vi "FGV_SerialControl.vi"(0 "Action":T1=enum."Close Serial Port", 1 "VISA Refnum in":refnum<visa-resource-name>="COM6", 2 "Channel":u8=255 step=1, 3 "Voltage":dbl min=0.0 max=4095.0 step=1.0, 4 "Wait Time (ms)":u32=4) -> (7 "VISA Refnum out":refnum<visa-resource-name>, 8 "Channels":u8[](array[numeric]), 9 "Voltages":u16[](array[numeric]), 10 "error out":errorcluster={"status"=FALSE, "code"=1073676294, "source"="VISA Read in SVI_ReadFromArduino.vi->FGV_SerialControl.vi->DemoForLoopWriteRead.vi"})   [LabVIEW 2020]
uses:
  Typedef_SerialFGVActions.ctl
  <vilib>/Instr/_visa.llb/VISA Configure Serial Port (Instr).vi
panel:
  out "Connection time (ms)":u32=1460
  out "read buffer":string="Connected\r\n"
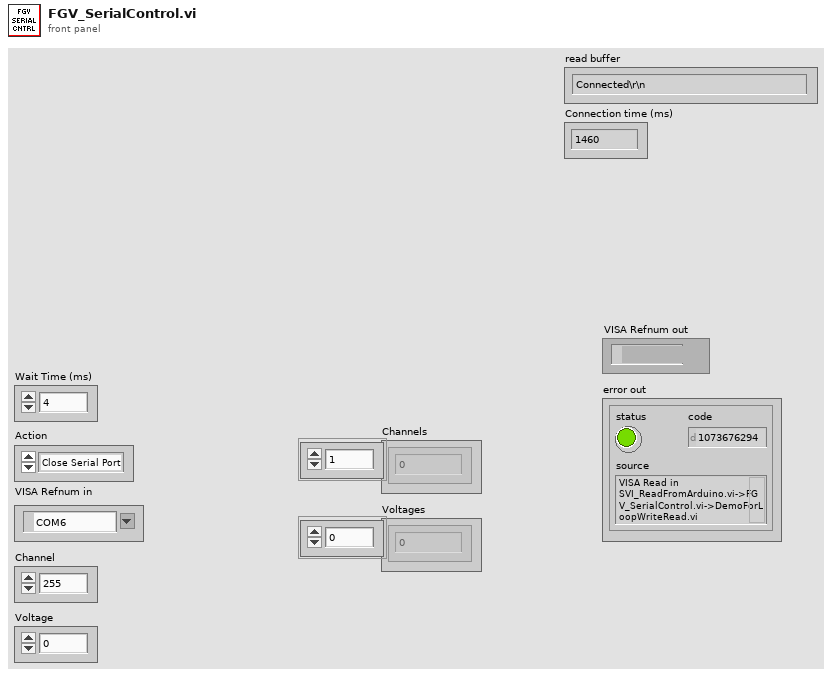
[diagram p1: front panel]
types:
  T1 = typedef "Typedef_SerialFGVActions.ctl" = enum16{"Open Serial Port", "Close Serial Port", "Update DAC", "Read ADC", "Read All ADCs"}
  T2 = cluster{"baud rate":u32, "data bits":u16, "parity":enum16{"None", "Odd", "Even", "Mark", "Space"}, "stop bits":u16, "flow control":u16}
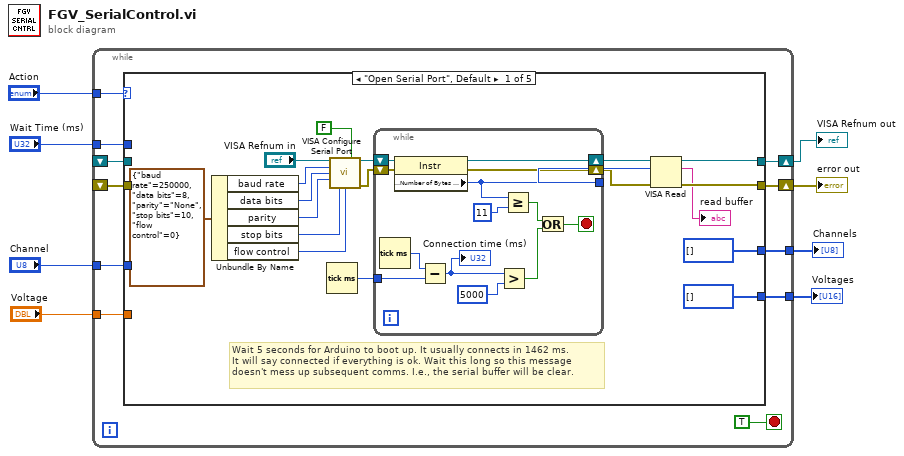
[diagram p0: block diagram]
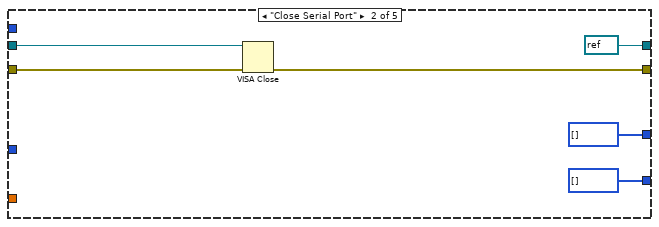
[diagram p2: hidden frame]
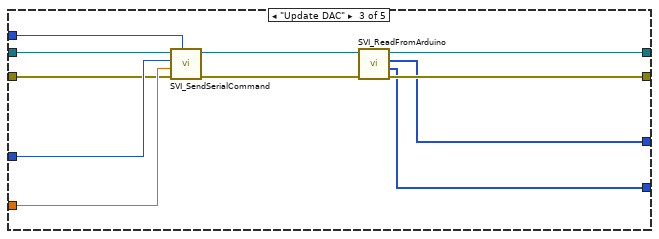
[diagram p3: hidden frame]
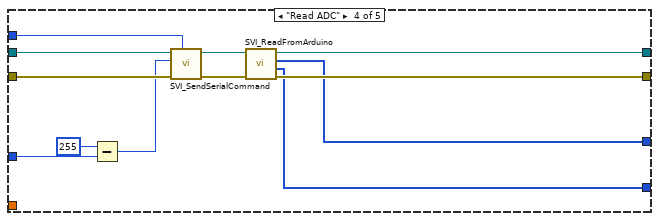
[diagram p4: hidden frame]
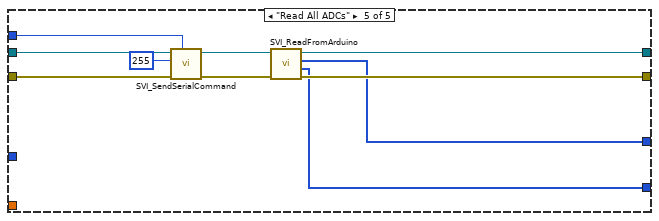
[diagram p5: hidden frame]
diagram:
  n1 = while {
    tunnel: "Action" -> [w19]
    shift-right: [w18] -> w6
    shift-left: _ -> [w16]
    shift-right: [w17] -> w7
    shift-left: _ -> [w15]
    tunnel: "Channel" -> [w14]
    tunnel: "Voltage" -> [w13]
    tunnel: [w12] -> w3
    tunnel: [w11] -> w2
    tunnel: "Wait Time (ms)" -> [w9]
    stop <- TRUE stop-if-true
    n2 = case shown="\"Open Serial Port\", Default" w19 {
      tunnel: [w26 refnum<visa-resource-name> refnum ("VISA Refnum out") w61 w75 w87] -> w18
      tunnel: [w25 w55 w62 w76 w86] -> w17
      tunnel: w16 -> [_ w57 w65 w79 w89]
      tunnel: w15 -> [_ w56 w66 w80 w90]
      tunnel: w14 -> [_ _ w68 w71 _]
      tunnel: w13 -> [_ _ w67 _ _]
      tunnel: [u16[] [] ("Voltages") u16[] [] ("Voltages") w60 w73 w83] -> w12
      tunnel: [u8[] [] ("Channels") u8[] [] ("Channels") w59 w74 w82] -> w11
      tunnel: w9 -> [_ _ w58 w72 w81]
      frame "Open Serial Port", Default {
        # "Wait 5 seconds for Arduino to boot up. It usually connects in 1462 ms. \nIt will say connected if everything is ok. Wait this long so this message\ndoesn't mess up subsequent comms. I.e., the serial buffer will be clear."
        n3 = Unbundle By Name(T2 {"baud rate"=250000, "data bits"=8, "parity"=enum."None", "stop bits"=10, "flow control"=0} ("Serial Settings")) -> ("baud rate"=w37:u32, "data bits"=w36:u16, "parity"=w35:enum16{"None", "Odd", "Even", "Mark", "Space"}, "stop bits"=w34:u16, "flow control"=w33:u16)
        n4 = Tick Count (ms)() -> (millisecond timer value=w21:u32)
        n5 = call-poly "VISA Configure Serial Port"("VISA resource name"="VISA Refnum in", "Enable Termination\nChar (T)"=FALSE ("Enable Termination\nChar (T)"), "baud rate (9600)"=w37, "data bits (8)"=w36, "parity (0:none)"=w35, "stop bits (10: 1 bit)"=w34, "flow control (0:none)"=w33) -> ("VISA resource name out"=w22:refnum<visa-resource-name>, "error out"=w23:errorcluster)  [unwired: 2 in, 5 out]
        n6 = while {
          tunnel: [w47] -> w29
          shift-right: [w51] -> w28
          shift-left: w23 -> [w49]
          shift-right: [w50] -> w27
          shift-left: w22 -> [w48]
          tunnel: w21 -> [w42]
          stop <- w44 stop-if-true
          n7 = Tick Count (ms)() -> (millisecond timer value=w43:u32)
          n8 = property class="Instr"(reference=w48, error in=w49) -> (reference out=w50:refnum<visa-resource-name>, error out=w51:errorcluster, "Serial Settings:Number of Bytes at Serial Port"=w47:u32)
          n9 = Subtract(x=w43, y=w42) -> (x-y=w41:u32)
          "Connection time (ms)" <- w41
          n10 = Greater?(x=w41, y=u32 5000) -> (0:w39:bool)
          n11 = Greater Or Equal?(x=w47, y=u32 11) -> (x >= y?=w45:bool)
          n12 = Or(x=w45, y=w39) -> (x .or. y?=w44:bool)
        }
        n13 = VISA Read(VISA resource name=w27, byte count=w29, error in (no error)=w28) -> (VISA resource name out=w26:refnum<visa-resource-name>, read buffer=→"read buffer":string, error out=w25:errorcluster)  [unwired: 1 out]
      }
      frame "Close Serial Port" {
        n14 = VISA Close(VISA resource name=w57, error in (no error)=w56) -> (error out=w55:errorcluster)
      }
      frame "Update DAC" {
        n15 = call "SVI_SendSerialCommand.vi"("Poll Time (ms)"=w58, "error in (no error)"=w66, "Voltage"=w67, "Channel"=w68, "VISA Refnum in"=w65) -> ("error out"=w64:errorcluster, "VISA Refnum out"=w63:refnum<visa-resource-name>)  [unwired: 5 in]
        n16 = call "SVI_ReadFromArduino.vi"("error in (no error)"=w64, "VISA Refnum in"=w63) -> ("error out"=w62:errorcluster, "Voltages"=w60:u16[], "Channels"=w59:u8[], "VISA Refnum out"=w61:refnum<visa-resource-name>)  [unwired: 6 in]
      }
      frame "Read ADC" {
        n17 = Subtract(x=u8 255, y=w71) -> (x-y=w69:u8)
        n18 = call "SVI_SendSerialCommand.vi"("Poll Time (ms)"=w72, "error in (no error)"=w80, "Channel"=w69, "VISA Refnum in"=w79) -> ("error out"=w78:errorcluster, "VISA Refnum out"=w77:refnum<visa-resource-name>)  [unwired: 6 in]
        n19 = call "SVI_ReadFromArduino.vi"("error in (no error)"=w78, "VISA Refnum in"=w77) -> ("error out"=w76:errorcluster, "Voltages"=w73:u16[], "Channels"=w74:u8[], "VISA Refnum out"=w75:refnum<visa-resource-name>)  [unwired: 6 in]
      }
      frame "Read All ADCs" {
        n20 = call "SVI_SendSerialCommand.vi"("Poll Time (ms)"=w81, "error in (no error)"=w90, "Channel"=u8 255 ("number"), "VISA Refnum in"=w89) -> ("error out"=w84:errorcluster, "VISA Refnum out"=w85:refnum<visa-resource-name>)  [unwired: 6 in]
        n21 = call "SVI_ReadFromArduino.vi"("error in (no error)"=w84, "VISA Refnum in"=w85) -> ("error out"=w86:errorcluster, "Voltages"=w83:u16[], "Channels"=w82:u8[], "VISA Refnum out"=w87:refnum<visa-resource-name>)  [unwired: 6 in]
      }
    }
  }
  "VISA Refnum out" <- w6
  "error out" <- w7
  "Channels" <- w2
  "Voltages" <- w3
